vi "Initialize Incoming.vi"(8 "error in (no error)":errorcluster, 10 "RT Configuration In":T1={"Name"="", "Priority"=100, "XNET Settings"={"Database"="", "Cluster"="", "Port"="", "Baud rate [Bd]"=0, "Termination"=0, "CAN I/O Mode"=0, "FD Baud rate [Bd]"=500000, "Priority"=100, "Use Legacy"=FALSE, "FD ISO Mode"=0}, "FPGA Session"=0, "Outgoing CAN Session"="", "Outgoing Frame Count"=0, "Outgoing Frames"=[], "Incoming CAN Session"="", "Incoming Frame Count"=0, "Incoming Frames"=[], "Incoming Values"={"Signal Values"=[], "Signal Invalid Values"=[], "ProtCtr Sig Values"=[], "Timestamps"=[], "Time Differences"=[], "IDs"=[]}} {"Incoming Frames"."Protection Configurations"."CRC Channels"."Data Type" items=["Signed", "Unsigned", "IEEE Float"]; "XNET Settings"."FD ISO Mode" items=["ISO", "Non ISO", "ISO Legacy"]; "XNET Settings"."CAN I/O Mode" items=["CAN 2.0", "CAN FD", "CAN FD+BRS"]; "XNET Settings"."Termination" items=["Off", "On"]; "Outgoing Frames"."Protection Configurations"."CRC Channels"."Data Type" items=["Signed", "Unsigned", "IEEE Float"]}, 11 "OnCompile Variables":T11={"Name"="", "XNET Settings"={"Database"="", "Cluster"="", "Port"="", "Baud rate [Bd]"=500000, "Termination"=1, "CAN I/O Mode"=0, "FD Baud rate [Bd]"=500000, "Priority"=100, "Use Legacy"=FALSE, "FD ISO Mode"=0}, "Frames"=[], "986x Support"={"Enable"=FALSE, "RIO Device"="", "Bitfile"=path ""}, "Incoming Frames"=[]} {"Incoming Frames"."Protection Configurations"."CRC Channels"."Data Type" items=["Signed", "Unsigned", "IEEE Float"]; "XNET Settings"."FD ISO Mode" items=["ISO", "Non ISO", "ISO Legacy"]; "XNET Settings"."CAN I/O Mode" items=["CAN 2.0", "CAN FD", "CAN FD+BRS"]; "XNET Settings"."Termination" items=["Off", "On"]; "Frames"."Protection Configurations"."CRC Channels"."Data Type" items=["Signed", "Unsigned", "IEEE Float"]}) -> (0 "error out":errorcluster, 3 "RT Configuration Out":T1={"Name"="", "Priority"=100, "XNET Settings"={"Database"="", "Cluster"="", "Port"="", "Baud rate [Bd]"=0, "Termination"=0, "CAN I/O Mode"=0, "FD Baud rate [Bd]"=500000, "Priority"=100, "Use Legacy"=FALSE, "FD ISO Mode"=0}, "FPGA Session"=0, "Outgoing CAN Session"="", "Outgoing Frame Count"=0, "Outgoing Frames"=[], "Incoming CAN Session"="", "Incoming Frame Count"=0, "Incoming Frames"=[], "Incoming Values"={"Signal Values"=[], "Signal Invalid Values"=[], "ProtCtr Sig Values"=[], "Timestamps"=[], "Time Differences"=[], "IDs"=[]}} {"Incoming Frames"."Protection Configurations"."CRC Channels"."Data Type" items=["Signed", "Unsigned", "IEEE Float"]; "XNET Settings"."FD ISO Mode" items=["ISO", "Non ISO", "ISO Legacy"]; "XNET Settings"."CAN I/O Mode" items=["CAN 2.0", "CAN FD", "CAN FD+BRS"]; "XNET Settings"."Termination" items=["Off", "On"]; "Outgoing Frames"."Protection Configurations"."CRC Channels"."Data Type" items=["Signed", "Unsigned", "IEEE Float"]})   [LabVIEW 2019, in "Ghost Bus Addon Engine.lvlib"]
uses:
  Ghost Bus Addon Engine.lvlib
  Addon Shared/Types/Exported.OnCompile.ctl
  Addon Shared/Types/XNET Settings.ctl
  SubModules/Frame-Protection-Support/Source/Shared/Types/Exported Frame Settings.ctl
  SubModules/Frame-Protection-Support/Source/Shared/Types/Exported Frame Type.ctl
  SubModules/Frame-Protection-Support/Source/Shared/Types/Exported Protection Settings.ctl
  SubModules/Frame-Protection-Support/Source/Shared/Types/Protection Type.ctl
  SubModules/Frame-Protection-Support/Source/Shared/Types/XNET Signal Configuration.ctl
  SubModules/Frame-Protection-Support/Source/Shared/Types/Exported Counter Settings.ctl
  SubModules/Frame-Protection-Support/Source/Shared/Types/Exported Event Trigger Type.ctl
  Addon Shared/Types/986x.ctl
  Types/RT Async Engine Settings.ctl
  SubModules/Frame-Protection-Support/Source/Engine/Types/RT Frame Settings.ctl
  SubModules/Frame-Protection-Support/Source/Engine/Types/RT Protection Configuration.ctl
  SubModules/Frame-Protection-Support/Source/Engine/Types/RT Frame Incoming Values.ctl
  <vilib>/xnet/xnet.llb/XNET Create Session (Frame Input Stream).vi
  <resource>/objmgr/xnet.rc
  SubModules/Frame-Protection-Support/Source/Engine/Protection and Counter Support Engine.lvlib
  SubModules/Frame-Protection-Support/Source/Shared/Protection and Counter Support Shared.lvlib
  Addon Shared/Ghost Bus Addon Shared.lvlib
panel:
  in  "PCL (usec)":u32
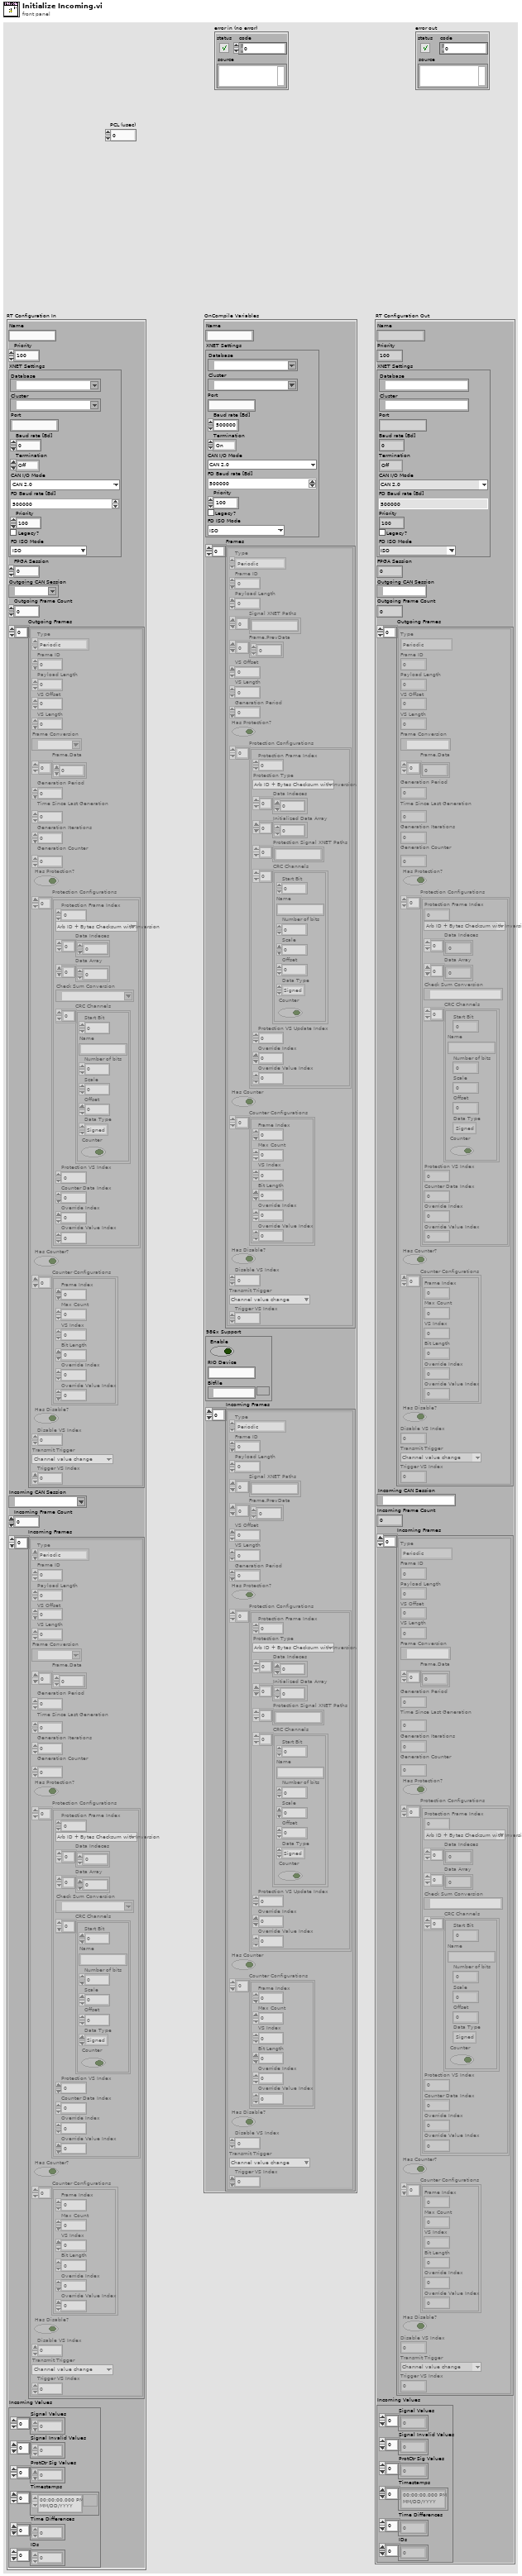
[diagram p1: front panel]
types:
  T1 = typedef "Ghost Bus Addon Engine.lvlib/RT Async Engine Settings.ctl" = cluster{"Name":string, "Priority":i32, "XNET Settings":T2, "FPGA Session":u32, "Outgoing CAN Session":refnum<k21>, "Outgoing Frame Count":i32, "Outgoing Frames":T3[], "Incoming CAN Session":refnum<k21>, "Incoming Frame Count":i32, "Incoming Frames":T3[], "Incoming Values":T10}
  T2 = typedef "Ghost Bus Addon Shared.lvlib/XNET Settings.ctl" = cluster{"Database":refnum<k21>, "Cluster":refnum<k21>, "Port":string, "Baud rate [Bd]":u64, "Termination":u32, "CAN I/O Mode":u32, "FD Baud rate [Bd]":u64, "Priority":i32, "Use Legacy":bool, "FD ISO Mode":u32}
  T3 = typedef "Protection and Counter Support Engine.lvlib/RT Frame Settings.ctl" = cluster{"Type":T4, "Frame ID":u32, "Payload Length":u32, "VS Offset":i32, "VS Length":i32, "Frame Conversion":refnum<k21>, "Frame.Data":dbl[], "Generation Period":u32, "Time Since Last Generation":u32, "Generation Iterations":u32, "Generation Counter":u32, "Has Protection?":bool, "Protection Configurations":T5[], "Has Counter?":bool, "Counter Configurations":T8[], "Has Disable?":bool, "Disable VS Index":i32, "Transmit Trigger":T9, "Trigger VS Index":i32}
  T4 = typedef "Protection and Counter Support Shared.lvlib/Exported Frame Type.ctl" = enum16{"Periodic", "Event", "Periodic/Event"}
  T5 = typedef "Protection and Counter Support Engine.lvlib/RT Protection Configuration.ctl" = cluster{"Protection Frame Index":i32, "Protection Type":T6, "Data Indeces":i32[], "Data Array":dbl[], "Check Sum Conversion":refnum<k21>, "CRC Channels":T7[], "Protection VS Index":i32, "Counter Data Index":i32, "Override Index":i32, "Override Value Index":i32}
  T6 = typedef "Protection and Counter Support Shared.lvlib/Protection Type.ctl" = enum16{"Arb ID + Bytes Checksum with Inversion", "Arb ID + Bytes CRC with Inversion", "Reversed Raw Signal Checksum with Inversion", "Concatenated Two's Compliment"}
  T7 = typedef "Protection and Counter Support Shared.lvlib/XNET Signal Configuration.ctl" = cluster{"Start Bit":i32, "Name":string, "Number of bits":i32, "Scale":dbl, "Offset":dbl, "Data Type":u32, "Counter":bool}
  T8 = typedef "Protection and Counter Support Shared.lvlib/Exported Counter Settings.ctl" = cluster{"Frame Index":i32, "Max Count":dbl, "VS Index":i32, "Bit Length":i64, "Override Index":i32, "Override Value Index":i32}
  T9 = typedef "Protection and Counter Support Shared.lvlib/Exported Event Trigger Type.ctl" = enum16{"Channel value change", "Trigger channel (not zero)", "Channel value change or trigger channel (not zero)", "Trigger channel (any value change)", "Channel value change or trigger channel (any value change)"}
  T10 = typedef "Protection and Counter Support Engine.lvlib/RT Frame Incoming Values.ctl" = cluster{"Signal Values":dbl[], "Signal Invalid Values":dbl[], "ProtCtr Sig Values":dbl[], "Timestamps":timestamp[], "Time Differences":dbl[], "IDs":u32[]}
  T11 = typedef "Ghost Bus Addon Shared.lvlib/Exported.OnCompile.ctl" = cluster{"Name":string, "XNET Settings":T2, "Frames":T12[], "986x Support":T14, "Incoming Frames":T12[]}
  T12 = typedef "Protection and Counter Support Shared.lvlib/Exported Frame Settings.ctl" = cluster{"Type":T4, "Frame ID":u32, "Payload Length":u32, "Signal XNET Paths":string[], "Frame.PrevData":dbl[], "VS Offset":i32, "VS Length":i32, "Generation Period":u32, "Has Protection?":bool, "Protection Configurations":T13[], "Has Counter":bool, "Counter Configurations":T8[], "Has Disable?":bool, "Disable VS Index":i32, "Transmit Trigger":T9, "Trigger VS Index":i32}
  T13 = typedef "Protection and Counter Support Shared.lvlib/Exported Protection Settings.ctl" = cluster{"Protection Frame Index":i32, "Protection Type":T6, "Data Indeces":i32[], "Initialized Data Array":dbl[], "Protection Signal XNET Paths":string[], "CRC Channels":T7[], "Protection VS Update Index":i32, "Override Index":i32, "Override Value Index":i32}
  T14 = typedef "Ghost Bus Addon Shared.lvlib/986x.ctl" = cluster{"Enable":bool, "RIO Device":string, "Bitfile":path}
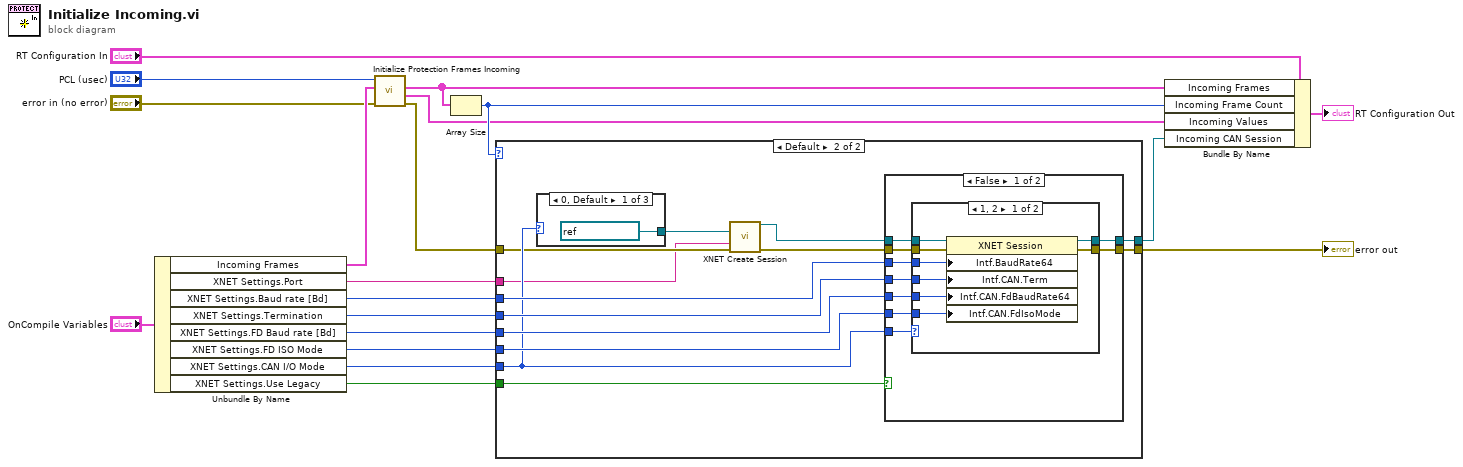
[diagram p0: block diagram]
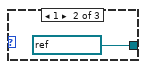
[diagram p3: hidden frame]
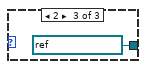
[diagram p4: hidden frame]
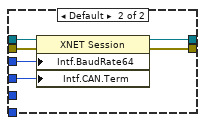
[diagram p5: hidden frame]
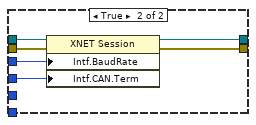
[diagram p6: hidden frame]
diagram:
  n1 = Unbundle By Name("OnCompile Variables") -> ("Incoming Frames"=w6:T12[], "XNET Settings.Port"=w9:string, "XNET Settings.Baud rate [Bd]"=w15:u64, "XNET Settings.Termination"=w16:u32, "XNET Settings.FD Baud rate [Bd]"=w17:u64, "XNET Settings.FD ISO Mode"=w12:u32, "XNET Settings.CAN I/O Mode"=w11:u32, "XNET Settings.Use Legacy"=w14:bool)
  n2 = call "Initialize Protection Frames Incoming.vi"("error in (no error)"="error in (no error)", "Frames"=w6, "PCL (usec)"="PCL (usec)") -> ("error out"=w2:errorcluster, "Frame Values"=w1:T10, "RT Frames"=w4:T3[])  [unwired: 6 in]
  n3 = Array Size(array=w4) -> (size(s)=w7:i32)
  n4 = case shown="Default" w7 {
    tunnel: w17 -> [_ w32]
    tunnel: w16 -> [_ w31]
    tunnel: w15 -> [_ w30]
    tunnel: w14 -> [_ w29]
    tunnel: [_ w28] -> w13
    tunnel: w12 -> [_ w26]
    tunnel: w11 -> [_ w25]
    tunnel: w2 -> [w20 w23]
    tunnel: w9 -> [_ w22]
    tunnel: [w20 w21] -> w8
    frame 0 {
      # "No incoming so ignore."
    }
    frame Default {
      n5 = case shown="0, Default" w25 {
        tunnel: [refnum<k21> ":memory:" ("cluster (:memory:)") refnum<k21> ":can_fd:" ("cluster (:memory:)") refnum<k21> ":can_fd_brs:" ("cluster (:memory:)")] -> w27
        frame 0, Default {
        }
        frame 1 {
        }
        frame 2 {
        }
      }
      n6 = call-poly <vilib>:"XNET Create Session.vi"("cluster (:memory:)"=w27, "interface"=w22, "error in (no error)"=w23) -> ("session out"=w33:refnum<k21>, "error out"=w24:errorcluster)  [unwired: 11 in]
      n7 = case shown="False" w29 {
        tunnel: w24 -> [w45 w65]
        tunnel: w33 -> [w44 w64]
        tunnel: [w43 w63] -> w21
        tunnel: w32 -> [w42 _]
        tunnel: w25 -> [w38 _]
        tunnel: w31 -> [w41 w60]
        tunnel: w30 -> [w40 w61]
        tunnel: [w39 w62] -> w28
        tunnel: w26 -> [w37 _]
        frame False {
          n8 = case shown="1, 2" w38 {
            tunnel: w45 -> [w53 w59]
            tunnel: w44 -> [w52 w58]
            tunnel: [w51 w57] -> w43
            tunnel: w42 -> [w50 _]
            tunnel: w41 -> [w49 w56]
            tunnel: w40 -> [w48 w55]
            tunnel: [w47 w54] -> w39
            tunnel: w37 -> [w46 _]
            frame 1, 2 {
              n9 = property class="XNET Session"(reference=w52, error in=w53, "Intf.BaudRate64"=w48, "Intf.CAN.Term"=w49, "Intf.CAN.FdBaudRate64"=w50, "Intf.CAN.FdIsoMode"=w46) -> (reference out=w47:refnum<k21>, error out=w51:errorcluster)
            }
            frame Default {
              n10 = property class="XNET Session"(reference=w58, error in=w59, "Intf.BaudRate64"=w55, "Intf.CAN.Term"=w56) -> (reference out=w54:refnum<k21>, error out=w57:errorcluster)
            }
          }
        }
        frame True {
          n11 = property class="XNET Session"(reference=w64, error in=w65, "Intf.BaudRate"=w61, "Intf.CAN.Term"=w60) -> (reference out=w62:refnum<k21>, error out=w63:errorcluster)
        }
      }
    }
  }
  "error out" <- w8
  n12 = Bundle By Name(cluster="RT Configuration In", "Incoming Frames"=w4, "Incoming Frame Count"=w7, "Incoming Values"=w1, "Incoming CAN Session"=w13) -> (→"RT Configuration Out":T1)
